vi "channels read.vi"(11 "Result Set (UTF-8)[2]":string) -> (3 "Array":string[](array[string]))   [LabVIEW 2020, in "Settings.lvlib"]
uses:
  Settings.lvlib
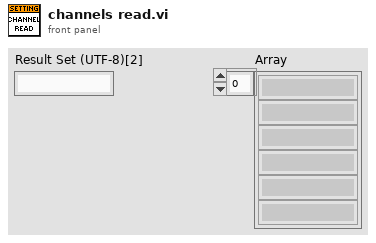
[diagram p1: front panel]
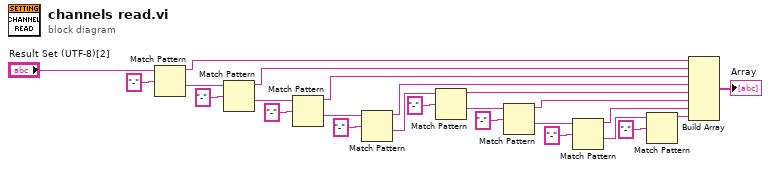
[diagram p0: block diagram]
diagram:
  n1 = Match Pattern(string="Result Set (UTF-8)[2]", regular expression="-") -> (before substring=w16:string, after substring=w8:string)  [unwired: 1 in, 2 out]
  n2 = Match Pattern(string=w8, regular expression="-") -> (before substring=w17:string, after substring=w7:string)  [unwired: 1 in, 2 out]
  n3 = Match Pattern(string=w7, regular expression="-") -> (before substring=w18:string, after substring=w5:string)  [unwired: 1 in, 2 out]
  n4 = Match Pattern(string=w5, regular expression="-") -> (before substring=w19:string, after substring=w3:string)  [unwired: 1 in, 2 out]
  n5 = Match Pattern(string=w3, regular expression="-") -> (before substring=w20:string, after substring=w12:string)  [unwired: 1 in, 2 out]
  n6 = Match Pattern(string=w12, regular expression="-") -> (before substring=w21:string, after substring=w14:string)  [unwired: 1 in, 2 out]
  n7 = Match Pattern(string=w14, regular expression="-") -> (before substring=w22:string, after substring=w24:string)  [unwired: 1 in, 2 out]
  n8 = Match Pattern(string=w24, regular expression="-") -> (before substring=w25:string)  [unwired: 1 in, 3 out]
  n9 = Build Array(w16, w17, w18, w19, w20, w21, w22, w25) -> (→"Array":string[])
